vi "Create.vi"(8 "error in (no error)":errorcluster, 11 "Plugin Manager in":refnum<class "CIFPluginManager.lvclass">) -> (0 "error out":errorcluster, 3 "Plugin Manager out":refnum<class "CIFPluginManager.lvclass">)   [LabVIEW 2021, in "CIFPluginManager.lvclass"]
uses:
  CIFPluginManager.lvclass
  CIFUtilities/CIFLogs/Typedef/Message Type.ctl
  <vilib>/CIF Foundation/CIF Utilities/Time/Typedef/Clock History Map.ctl
  <vilib>/CIF Foundation/CIF Utilities/Time/Typedef/Clock History.ctl
  <vilib>/CIF Foundation/CIF Utilities/Time/Typedef/Timestamp Pair.ctl
  typedef/Plugin Management Data Map.ctl
  typedef/Plugin Management Data.ctl
  <vilib>/gRPC/LabVIEW gRPC Library/Shared/grpcId.ctl
  typedef/Loader Type.ctl
  CIFCore/Common/Typedef/Version.ctl
  gRPC/CIF_Manager_server/RPC Messages/cif_plugincore_StatusData.ctl
  gRPC/CIF_Manager_server/RPC Messages/cif_plugincore_StatusData_PluginState.ctl
  gRPC/CIF_Manager_server/RPC Messages/cif_plugincore_TimingStatistics.ctl
  gRPC/CIF_Manager_server/RPC Messages/cif_common_TimingStats.ctl
  gRPC/CIF_Manager_server/RPC Messages/cif_plugincore_FifoStatistics.ctl
  gRPC/CIF_Manager_server/RPC Messages/cif_plugincore_Error.ctl
  gRPC/CIF_Manager_server/RPC Messages/cif_plugincore_MonitorDoubles.ctl
  gRPC/CIF_Manager_server/RPC Messages/cif_plugincore_MonitorU64.ctl
  gRPC/CIF_Manager_server/RPC Messages/cif_plugincore_MonitorI64.ctl
  gRPC/CIF_Manager_server/RPC Messages/cif_channelcore_Channels.ctl
  gRPC/CIF_Manager_server/RPC Messages/cif_channelcore_Channel.ctl
  gRPC/CIF_Manager_server/RPC Messages/cif_channelcore_ChannelDirection.ctl
  gRPC/CIF_Manager_server/RPC Messages/cif_channelcore_ChannelPattern.ctl
  typedef/Discovered Plugin Map.ctl
  typedef/Discovered Plugin.ctl
  typedef/Plugin Metadata.ctl
  typedef/Loader Map.ctl
  typedef/Loaders.ctl
  CIFPluginManager.lvclass/CIFPluginManager.ctl
  CIFUtilities/CIFConfigurationFile/CIF Configuration File.lvlib
  CIFUtilities/CIFLogs/CIFLogs.lvlib
  <vilib>/CIF Foundation/CIF Utilities/Time/Time_CIF_U.lvlib
  gRPC/CIF_Manager_server/CIF_Manager_server.lvlib
  CIFCore/Common/CIFCoreCommon.lvlib
  <vilib>/gRPC/LabVIEW gRPC Library/grpc-lvsupport-release.lvlib
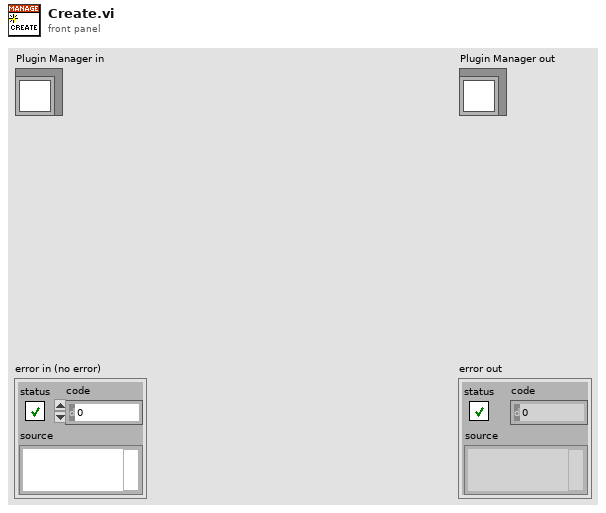
[diagram p1: front panel]
types:
  T1 = typedef "CIFPluginManager.lvclass/Loader Map.ctl" = map{string, T2}
  T2 = typedef "CIFPluginManager.lvclass/Loaders.ctl" = cluster{"Loader Type":T3, "grpc_port":i32, "pid":u32, "gRPC ID":T4, "Load Timestamp":i64, "Unloading":bool, "Ready for removal":bool, "Unload Timestamp":i64}
  T3 = typedef "CIFPluginManager.lvclass/Loader Type.ctl" = enum16{"LabVIEW"}
  T4 = typedef "grpc-lvsupport-release.lvlib/grpcId.ctl" = u64
  T5 = typedef "CIFPluginManager.lvclass/Discovered Plugin Map.ctl" = map{string, T6[]}
  T6 = typedef "CIFPluginManager.lvclass/Discovered Plugin.ctl" = cluster{"Filename":string, "Plugin Type":string, "Qualified name":string, "Version":T7, "Plugin Metadata":T8, "Loader Type":T3, "File Path":string, "Relative Path":string[]}
  T7 = typedef "CIFCoreCommon.lvlib/Version.ctl" = cluster{"Major":i32, "Minor":i32, "Fix":i32, "Build":i32}
  T8 = typedef "CIFPluginManager.lvclass/Plugin Metadata.ctl" = cluster{"Description":string, "History":string, "Author":string}
  T9 = typedef "CIFPluginManager.lvclass/Plugin Management Data Map.ctl" = map{string, T10}
  T10 = typedef "CIFPluginManager.lvclass/Plugin Management Data.ctl" = cluster{"Unique Name":string, "Plugin Type":string, "gRPC Port":i32, "gRPC ID":T4, "Loader Type":T3, "Loader":string, "Version":T7, "Load Timestamp":i64, "Unload Timestamp":i64, "Unloading":bool, "Ready for removal":bool, "status":T11, "channels":T20}
  T11 = typedef "CIF_Manager_server.lvlib/cif_plugincore_StatusData.ctl" = cluster{"state":T12, "timing_statistics":T13, "fifo_statistics":T15, "error":T16, "monitor_doubles":T17, "monitor_u64s":T18, "monitor_i64s":T19}
  T12 = typedef "CIF_Manager_server.lvlib/cif_plugincore_StatusData_PluginState.ctl" = enum32{"PLUGINSTATE_UNKNOWN", "PLUGINSTATE_CREATING", "PLUGINSTATE_LISTENING", "PLUGINSTATE_RUNNING", "PLUGINSTATE_CLEANINGUP", "PLUGINSTATE_DESTROYING"}
  T13 = typedef "CIF_Manager_server.lvlib/cif_plugincore_TimingStatistics.ctl" = cluster{"period":T14, "wake_error":T14, "execute":T14, "housekeep":T14, "idle":T14, "cleanup":T14, "custom_1":T14, "custom_2":T14}
  T14 = typedef "CIF_Manager_server.lvlib/cif_common_TimingStats.ctl" = cluster{"max":i64, "min":i64, "avg":dbl}
  T15 = typedef "CIF_Manager_server.lvlib/cif_plugincore_FifoStatistics.ctl" = cluster{"from_t0":T14, "from_previous_plugin":T14, "output_error":T14}
  T16 = typedef "CIF_Manager_server.lvlib/cif_plugincore_Error.ctl" = cluster{"status":bool, "code":i32}
  T17 = typedef "CIF_Manager_server.lvlib/cif_plugincore_MonitorDoubles.ctl" = cluster{"double_1":dbl, "double_2":dbl, "double_3":dbl, "double_4":dbl}
  T18 = typedef "CIF_Manager_server.lvlib/cif_plugincore_MonitorU64.ctl" = cluster{"u64_1":u64, "u64_2":u64, "u64_3":u64, "u64_4":u64}
  T19 = typedef "CIF_Manager_server.lvlib/cif_plugincore_MonitorI64.ctl" = cluster{"i64_1":i64, "i64_2":i64, "i64_3":i64, "i64_4":i64}
  T20 = typedef "CIF_Manager_server.lvlib/cif_channelcore_Channels.ctl" = cluster{"channels":T21[]}
  T21 = typedef "CIF_Manager_server.lvlib/cif_channelcore_Channel.ctl" = cluster{"name":string, "direction":T22, "type":string, "custom_config":u8[], "connected":bool, "connected_name":string, "forced":bool, "channel_pattern":T23}
  T22 = typedef "CIF_Manager_server.lvlib/cif_channelcore_ChannelDirection.ctl" = enum32{"CHANNELDIRECTION_UNKNOWN", "CHANNELDIRECTION_PUBLISHER", "CHANNELDIRECTION_SUBSCRIBER"}
  T23 = typedef "CIF_Manager_server.lvlib/cif_channelcore_ChannelPattern.ctl" = enum32{"CHANNELPATTERN_UNKNOWN", "CHANNELPATTERN_TAG", "CHANNELPATTERN_FIFO", "CHANNELPATTERN_MULTIFIFO", "CHANNELPATTERN_BACKPRESSUREFIFO"}
  T24 = typedef "Time_CIF_U.lvlib/Clock History Map.ctl" = map{u8, T25}
  T25 = typedef "Time_CIF_U.lvlib/Clock History.ctl" = cluster{"System Clock":i64[], "External Clock":i64[], "Last Reset Time":i64, "slope":dbl, "1/slope":dbl, "Offset Pair":T26, "Name":string}
  T26 = typedef "Time_CIF_U.lvlib/Timestamp Pair.ctl" = cluster{"System Time":i64, "External Time":i64}
  T27 = typedef "CIFLogs.lvlib/Message Type.ctl" = enum16{"Error", "Information", "Print Terminal", "Configuration"}
  T28 = typedef "CIFLogs.lvlib/Log Info.ctl" = cluster{"size (bytes)":i64, "Last Timestamp":string}
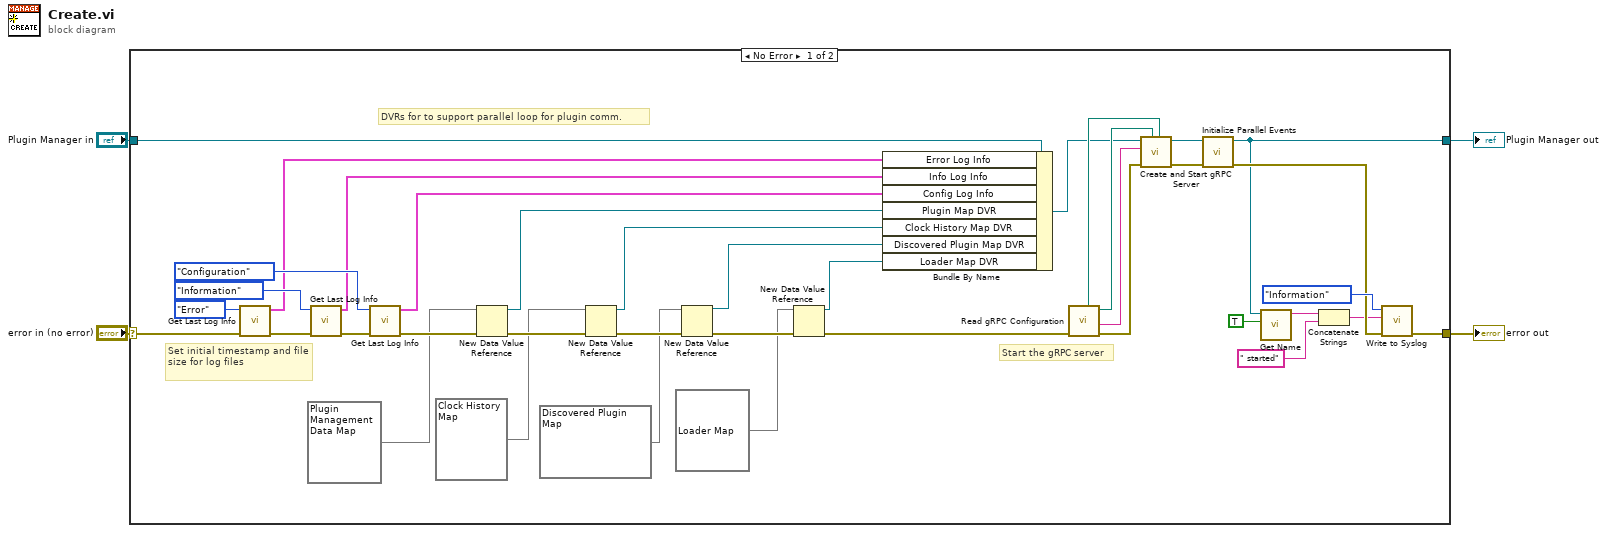
[diagram p0: block diagram]
diagram:
  n1 = case shown="No Error" "error in (no error)" {
    selector: "error in (no error)" -> [w32 w44]
    tunnel: [w33 w44] -> w3
    tunnel: [w6 w43] -> w1
    tunnel: "Plugin Manager in" -> [w38 w43]
    frame No Error {
      # "DVRs for to support parallel loop for plugin comm."
      # "Start the gRPC server"
      # "Set initial timestamp and file size for log files"
      n2 = call "Get Last Log Info.vi"("error in"=w32, "CIF Message Type"=Message_Type."Error") -> ("error out"=w30:errorcluster, "Log Info"=w24:T28)  [unwired: 8 in]
      n3 = call "Get Last Log Info.vi"("error in"=w30, "CIF Message Type"=Message_Type."Information") -> ("error out"=w27:errorcluster, "Log Info"=w25:T28)  [unwired: 8 in]
      n4 = call "Get Last Log Info.vi"("error in"=w27, "CIF Message Type"=Message_Type."Configuration") -> ("error out"=w23:errorcluster, "Log Info"=w26:T28)  [unwired: 8 in]
      n5 = New Data Value Reference(data value=T9 {} ("Plugin Map"), error in=w23) -> (data value reference=w22:refnum<data-value>, error out=w21:errorcluster)
      n6 = New Data Value Reference(data value=T24 {} ("Clock History Map"), error in=w21) -> (data value reference=w20:refnum<data-value>, error out=w16:errorcluster)
      n7 = New Data Value Reference(data value=T5 {} ("Discovered Plugins"), error in=w16) -> (data value reference=w14:refnum<data-value>, error out=w13:errorcluster)
      n8 = New Data Value Reference(data value=T1 {} ("map"), error in=w13) -> (data value reference=w10:refnum<data-value>, error out=w11:errorcluster)
      n9 = Bundle By Name(cluster=w38, "Error Log Info"=w24, "Info Log Info"=w25, "Config Log Info"=w26, "Plugin Map DVR"=w22, "Clock History Map DVR"=w20, "Discovered Plugin Map DVR"=w14, "Loader Map DVR"=w10) -> (w37:refnum<class "CIFPluginManager.lvclass">)
      n10 = call "Read gRPC Configuration.vi"("error in"=w11) -> ("error out"=w42:errorcluster, "Manager Server Address"=w39:string, "Server Certificate File (.crt)"=w40:path, "Server Key File (.key)"=w41:path)  [unwired: 5 in, 2 out]
      n11 = call "Create and Start gRPC Server.vi"("Server Key File (.key)"=w41, "Server Certificate File (.crt)"=w40, "error in (no error)"=w42, "Server Address"=w39, "Plugin Manager in"=w37) -> ("error out"=w35:errorcluster, "Plugin Manager out"=w36:refnum<class "CIFPluginManager.lvclass">)  [unwired: 5 in]
      n12 = call "Initialize Parallel Events.vi"("error in (no error)"=w35, "CIFPluginManager in"=w36) -> ("error out"=w17:errorcluster, "CIFPluginManager out"=w6:refnum<class "CIFPluginManager.lvclass">)  [unwired: 8 in]
      n13 = call "Get Name.vi"("Include Extra Info"=TRUE, "CIFPluginManager in"=w6) -> ("Name"=w9:string)  [unwired: 9 in]
      n14 = Concatenate Strings(w9, " started" ("message")) -> (w7:string)
      n15 = call "Write to Syslog.vi"("error in (no error)"=w17, "message"=w7, "CIF Message Type"=Message_Type."Information") -> ("error out"=w33:errorcluster)  [unwired: 8 in]
    }
    frame Error {
    }
  }
  "error out" <- w3
  "Plugin Manager out" <- w1
